vi "ManStatusPressureGaugeV2.vi"(8 "Error In":errorcluster, 11 "Show in":T1) -> (0 "Error Out":errorcluster, 3 "defect":bool)   [LabVIEW 2018]
uses:
  PressureGaugeInfo.ctl
panel:
  in  "Брак":bool
  in  "Установленно верно":bool
  out "message out":string caption="String"
  out "Manometr out":T2 {"MANOMETR" scale=0.0..2.5 scale format="%#.1f"}
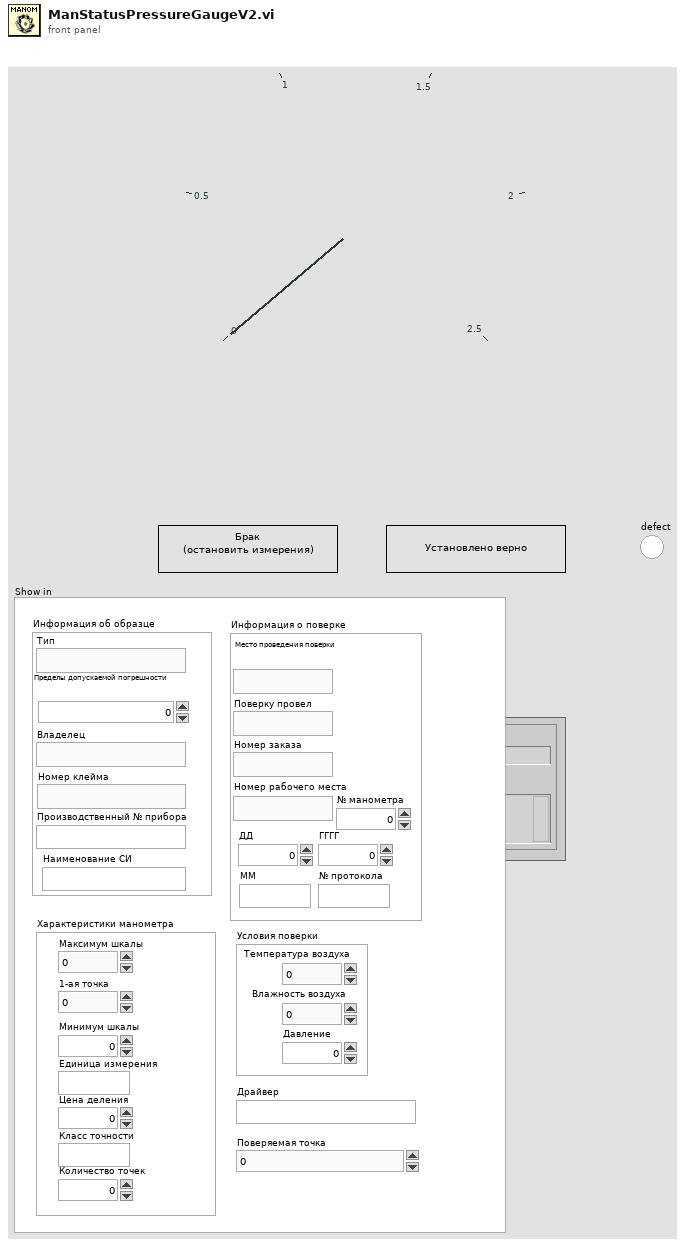
[diagram p1: front panel]
types:
  T1 = typedef "PressureGaugeInfo.ctl" = cluster{"Информация об образце":cluster{"Тип":string, "Владелец":string, "Номер клейма":string, "Пределы допускаемой погрешности ":dbl, "Производственный № прибора":string, "Наименование СИ":string}, "Информация о поверке":cluster{"Место проведения поверки":string, "Поверку провел":string, "Номер заказа":string, "Номер рабочего места":string, "ДД":dbl, "ММ":string, "ГГГГ":dbl, "№ протокола":string, "№ манометра":dbl}, "Характеристики манометра":cluster{"Максимум шкалы":dbl, "1-ая точка":dbl, "Единица измерения":string, "Цена деления":dbl, "Класс точности":string, "Минимум шкалы":dbl, "Количество точек":dbl}, "Условия поверки":cluster{"Температура воздуха":dbl, "Влажность воздуха":dbl, "Давление":dbl}, "Драйвер":string, "Поверяемая точка":dbl}
  T2 = cluster{"Единица измерения":string, "Класс точности":string, "Максимум шкалы":dbl, "MANOMETR":dbl}
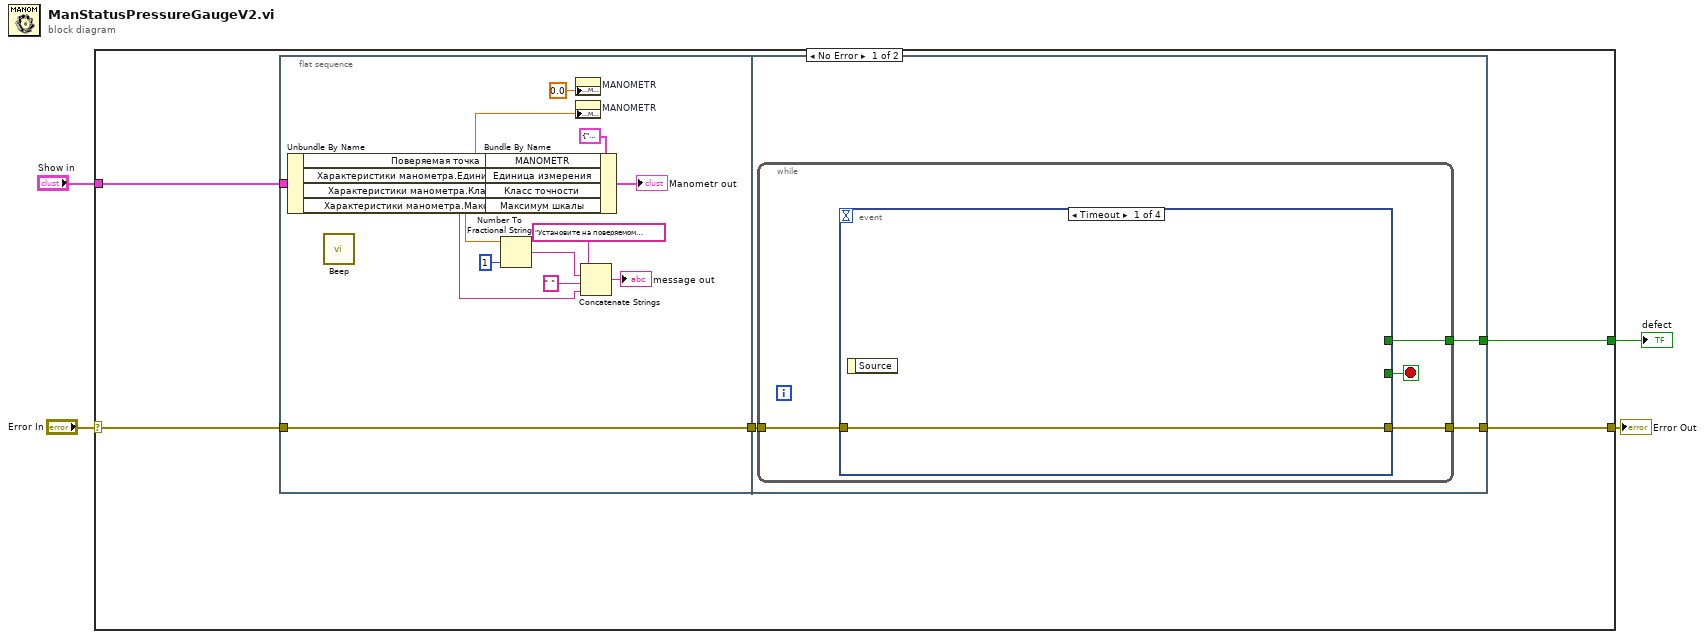
[diagram p0: block diagram]
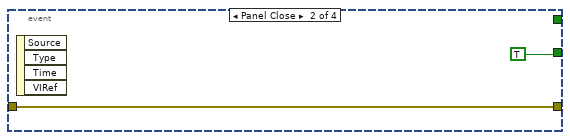
[diagram p2: hidden frame]
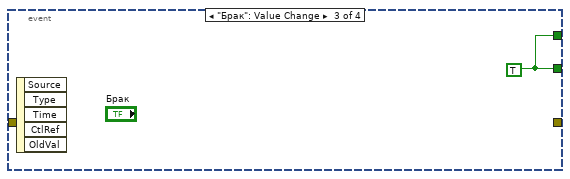
[diagram p3: hidden frame]
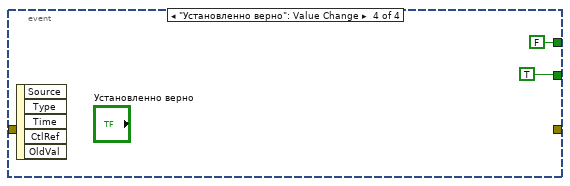
[diagram p4: hidden frame]
diagram:
  n1 = case shown="No Error" "Error In" {
    selector: "Error In" -> [w8 w37]
    tunnel: [w9 w37] -> w3
    tunnel: "Show in" -> [w6 _]
    tunnel: [w5 _] -> w1
    frame No Error {
      n2 = flat-sequence {
        tunnel: w8 -> [w23]
        tunnel: [w23] -> w7
        tunnel: w6 -> [w19]
        tunnel: [w26] -> w9
        tunnel: w7 -> [w25]
        tunnel: [w24] -> w5
        frame #0 {
          n3 = Unbundle By Name(w19) -> ("Поверяемая точка"=w11:dbl, "Характеристики манометра.Единица измерения"=w10:string, "Характеристики манометра.Класс точности"=w18:string, "Характеристики манометра.Максимум шкалы"=w17:dbl)
          n4 = call <vilib>:"Beep.vi"() -> ()  [unwired: 12 in]
          n5 = Bundle By Name(cluster=T2 {"Единица измерения"="", "Класс точности"="", "Максимум шкалы"=0.0, "MANOMETR"=0.0} ("Manometr out"), "MANOMETR"=w11, "Единица измерения"=w10, "Класс точности"=w18, "Максимум шкалы"=w17) -> (→"Manometr out":T2)
          n6 = Number To Fractional String(number=w11, precision (6)=i16 1) -> (F-format string=w16:string)  [unwired: 2 in]
          n7 = property on="MANOMETR" class="Knob (strict)"("Scale.Minimum"=0.0 ("Scale.Range:Minimum")) -> ()  [unwired: 2 in, 2 out]
          n8 = property on="MANOMETR" class="Knob (strict)"("Scale.Maximum"=w17) -> ()  [unwired: 2 in, 2 out]
          n9 = Concatenate Strings("Установите на поверяемом приборе давление " ("message in"), w16, " " ("string"), w10) -> (→"message out":string)
        }
        frame #1 {
          n10 = while {
            tunnel: [w29] -> w26
            tunnel: w25 -> [w28]
            tunnel: [w27] -> w24
            stop <- w30 stop-if-true
            n11 = event shown="[0] Timeout" {
              selector: _ -> [_ _ _ _]
              dyn-events: _ -> [_ _ _ _]
              timeout: _ -> [_ _ _ _]
              tunnel: [_ TRUE w34 TRUE] -> w30
              tunnel: [w31 w32 _ _] -> w29
              tunnel: w28 -> [w31 w32 _ _]
              tunnel: [_ _ w34 FALSE] -> w27
              event Timeout {
                n12 = event-data() -> ()  [unwired: 1 in, 1 out]
              }
              event Panel Close {
                n13 = event-data() -> ()  [unwired: 1 in, 4 out]
              }
              event "Брак": Value Change {
                w34 = TRUE
                n14 = event-data() -> ()  [unwired: 1 in, 5 out]
              }
              event "Установленно верно": Value Change {
                n15 = event-data() -> ()  [unwired: 1 in, 5 out]
              }
            }
          }
        }
      }
    }
    frame Error {
    }
  }
  "Error Out" <- w3
  "defect" <- w1
